vi "Tab_Num.vi"() -> ()   [LabVIEW 2020]
panel:
  out "Resul_tab 2":i32[][](array[numeric])
  out "tableau initialisé":i32[][](array[numeric])
  out "Resul_tab":i32[][](array[numeric])
  out "Indicateur Tab boucle":i32[][](array[numeric])
  in  "Tableau_int":u8[][](array[numeric])
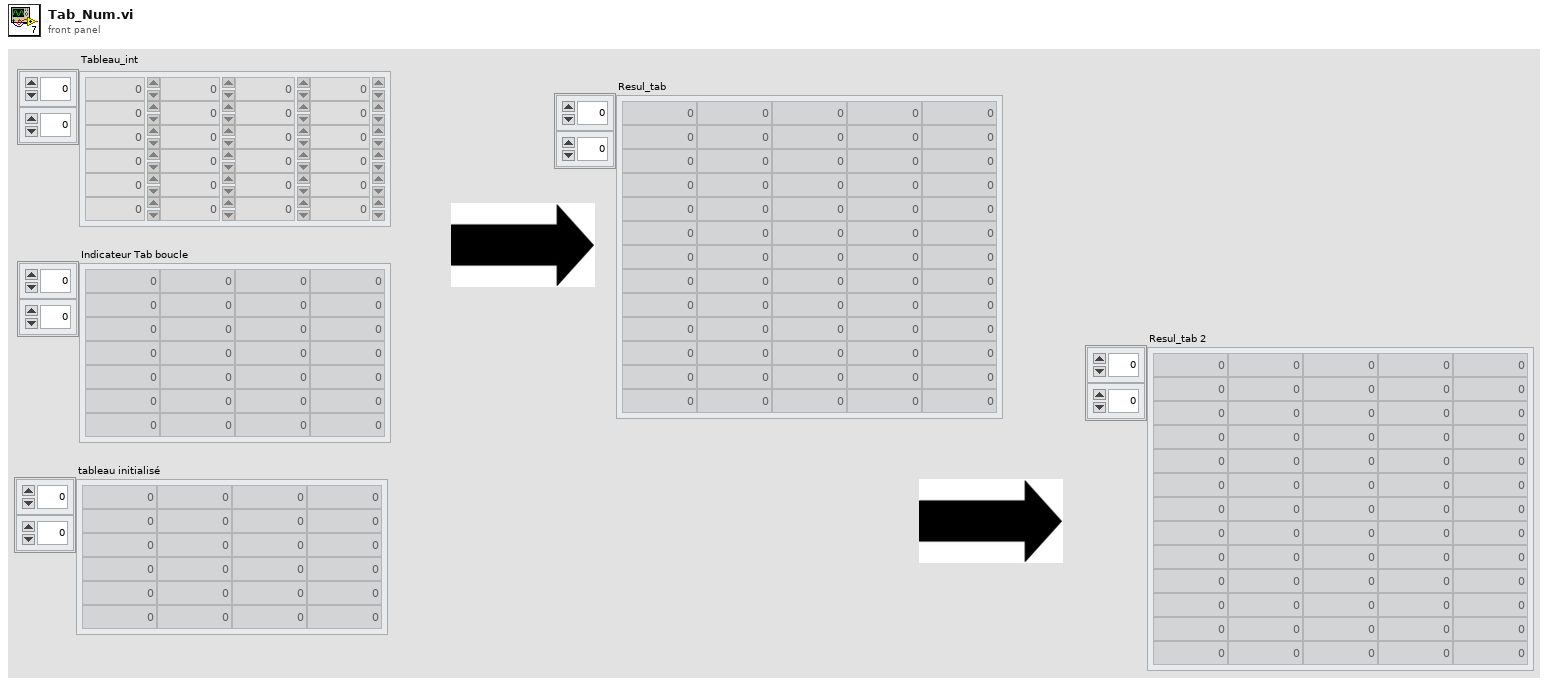
[diagram p1: front panel]
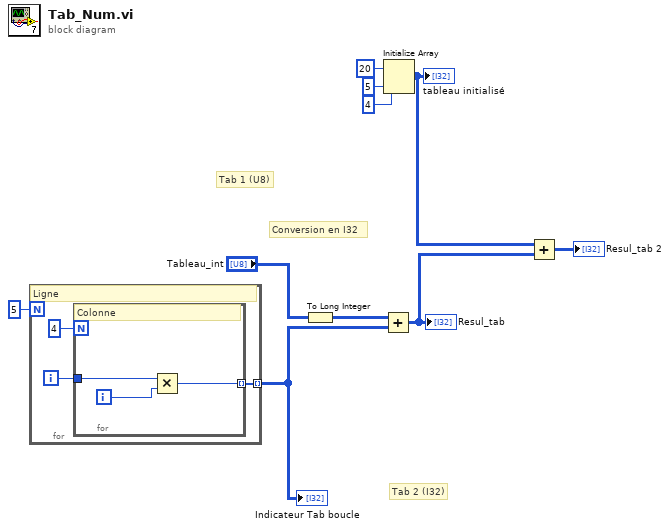
[diagram p0: block diagram]
diagram:
  # "Tab 2 (I32)"
  # "Tab 1 (U8)"
  # "Conversion en I32"
  n1 = for {
    N: 5 -> [_]
    tunnel: [w11] -> w8 mode=indexing
    i -> [w12]
    # "Ligne"
    n2 = for {
      N: 4 -> [_]
      tunnel: w12 -> [w16]
      tunnel: [w14] -> w11 mode=indexing
      i -> [w15]
      # "Colonne"
      n3 = Multiply(x=w16, y=w15) -> (x*y=w14:i32)
    }
  }
  "Indicateur Tab boucle" <- w8
  n4 = To Long Integer(number="Tableau_int") -> (32bit integer=w7:i32[][])
  n5 = Add(x=w7, y=w8) -> (x+y=w2:i32[][])
  "Resul_tab" <- w2
  n6 = Initialize Array(20 ("élément"), 5 ("taille de la dimension"), 4 ("taille de la dimension")) -> (w3:i32[][])
  "tableau initialisé" <- w3
  n7 = Add(x=w3, y=w2) -> (x+y=→"Resul_tab 2":i32[][])
